vi "motor_controller.vi"() -> ()   [LabVIEW 2020]
panel:
  in  "Crystal Number":u16(ring) items=["Crystal 1", "Crystal 2", "Crystal 3", "Crystal 4", "Crystal 5", "Crystal 6", "Crystal 7", ""]
  in  "Scan speed":dbl
  in  "End":dbl
  in  "Start":dbl
  in  "Start scan":bool
  in  "Tab Control":enum32{"Motor Controls", "Power"}(tab)
  in  "Motor 1":dbl
  in  "Motor 2":dbl
  in  "Motor 3":dbl
  in  "Motor 4":dbl
  in  "Motor 5":dbl
  in  "Motor 6":dbl
  in  "stop":bool
  in  "Motor 7":dbl
  in  "Movement speed":dbl
  in  "Step Size":dbl
  # "Motor Scan"
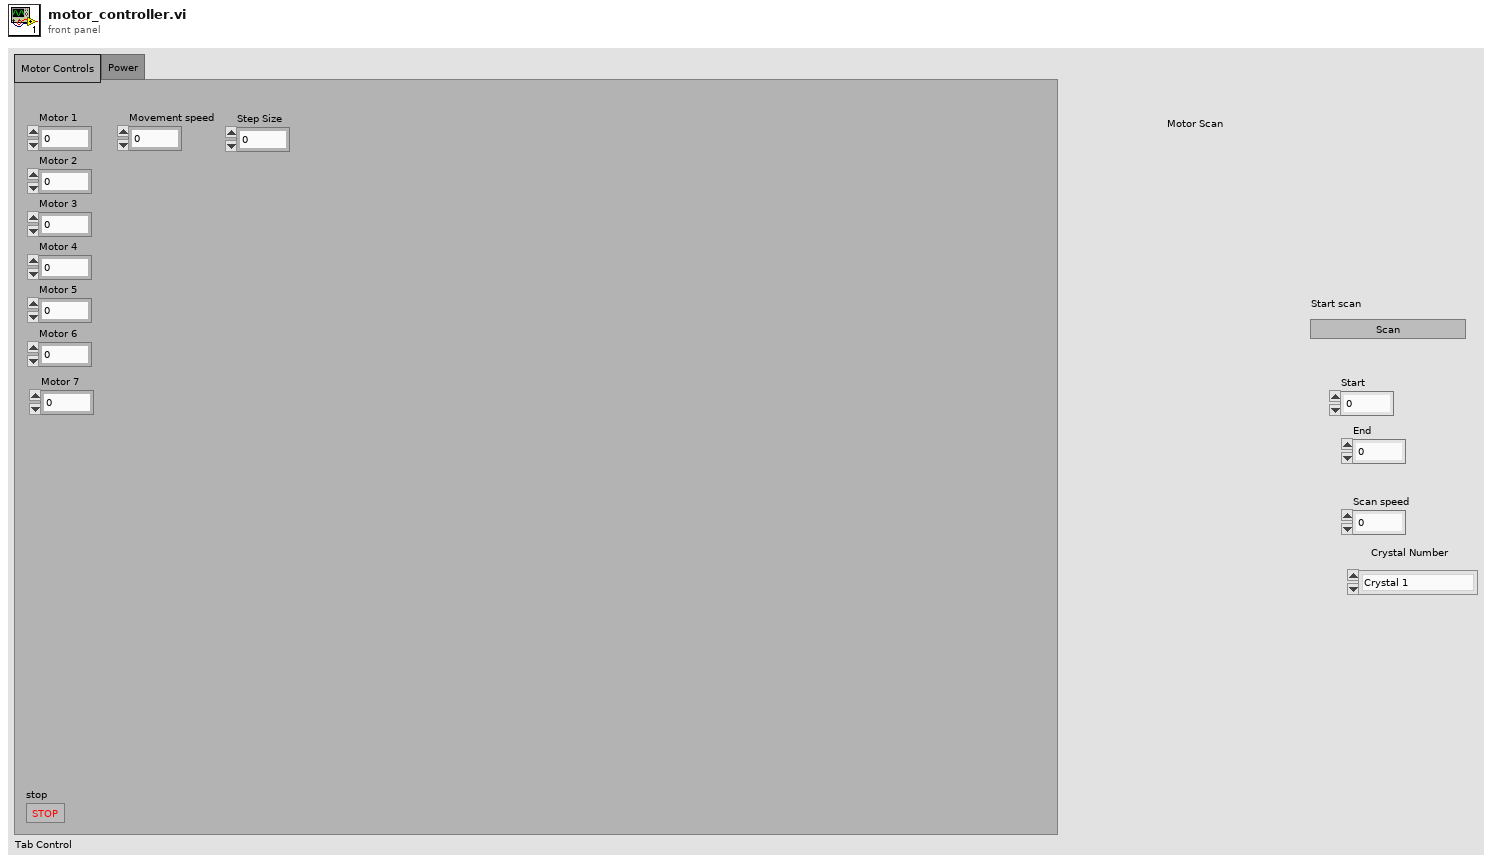
[diagram p1: front panel]
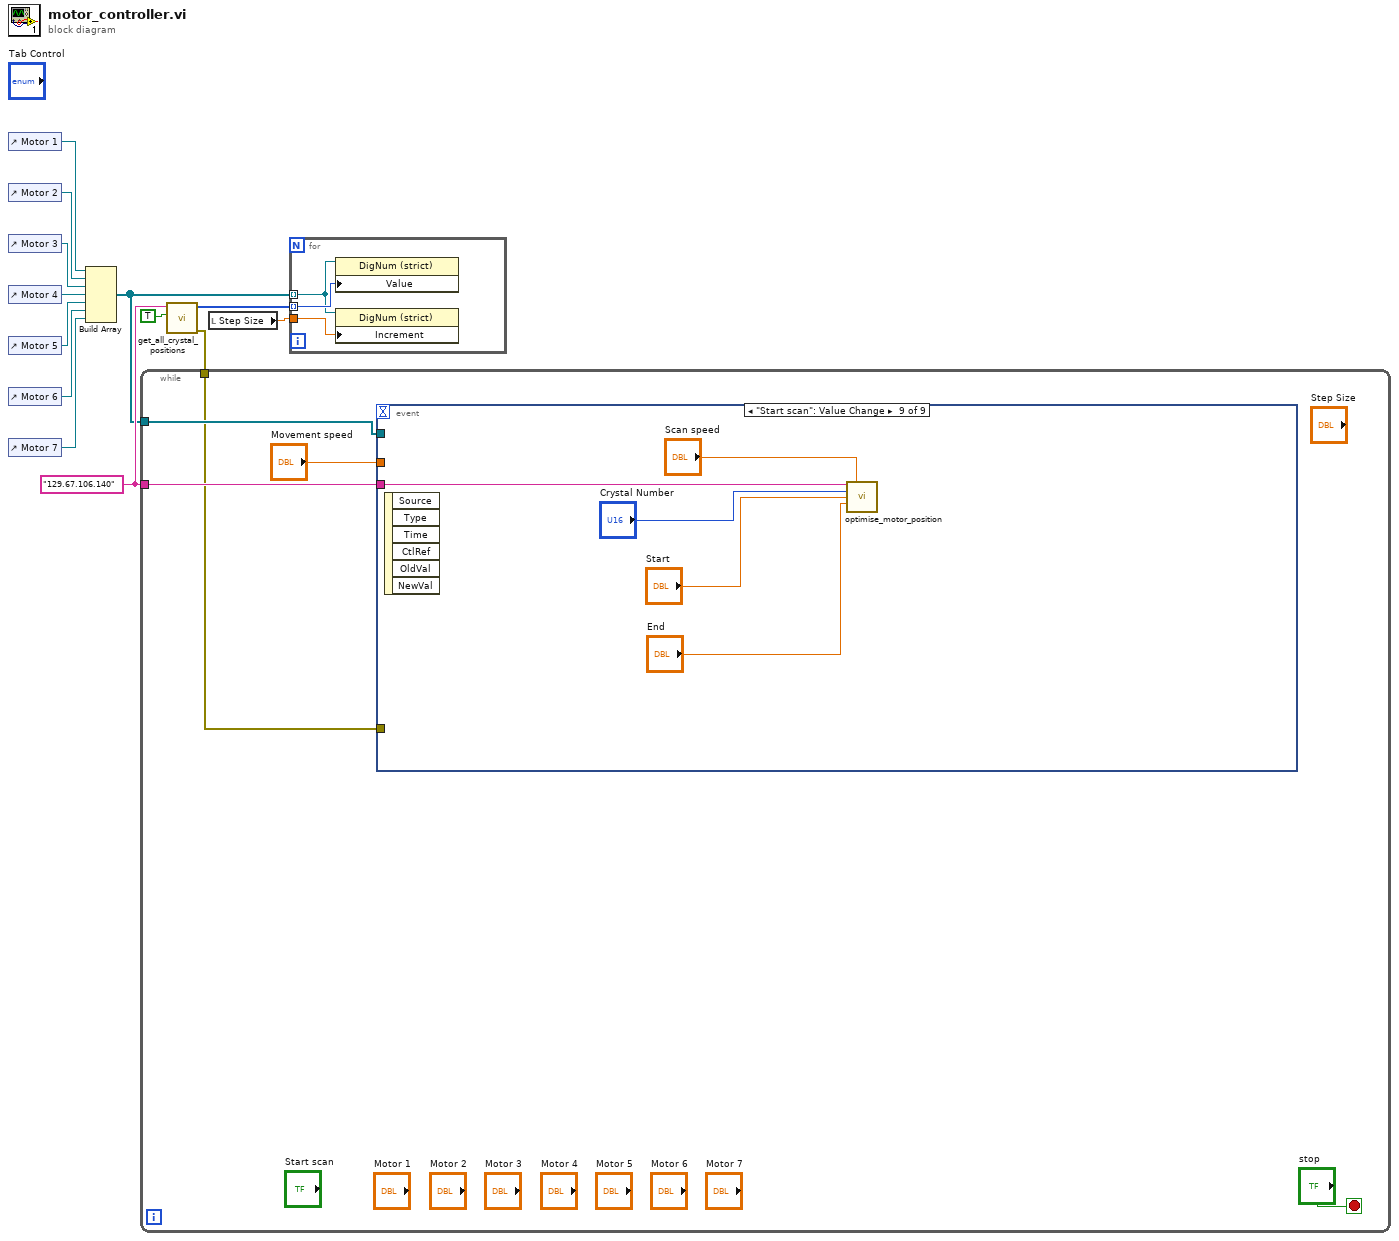
[diagram p0: block diagram]
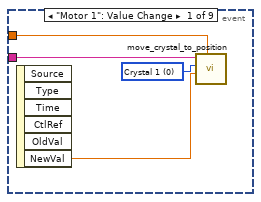
[diagram p2: hidden frame]
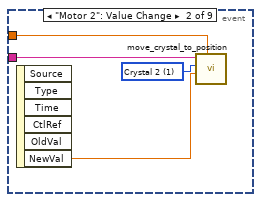
[diagram p3: hidden frame]
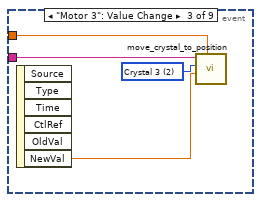
[diagram p4: hidden frame]
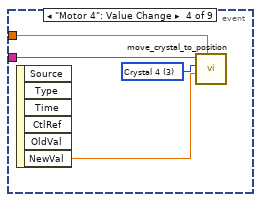
[diagram p5: hidden frame]
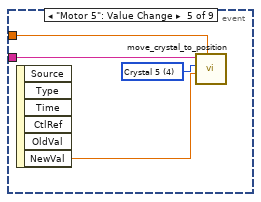
[diagram p6: hidden frame]
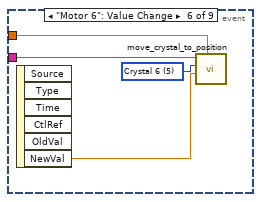
[diagram p7: hidden frame]
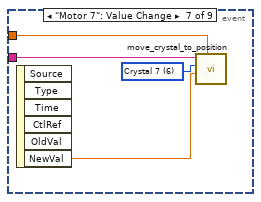
[diagram p8: hidden frame]
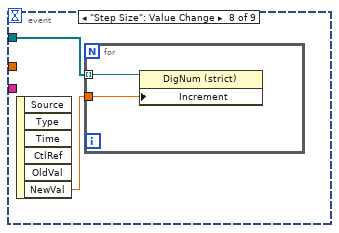
[diagram p9: hidden frame]
diagram:
  w4 = "129.67.106.140" ("address")
  n1 = control-ref of="Motor 1"() -> (w12:refnum<vi>)
  n2 = control-ref of="Motor 2"() -> (w11:refnum<vi>)
  n3 = control-ref of="Motor 3"() -> (w10:refnum<vi>)
  n4 = control-ref of="Motor 4"() -> (w9:refnum<vi>)
  n5 = control-ref of="Motor 5"() -> (w8:refnum<vi>)
  n6 = control-ref of="Motor 6"() -> (w7:refnum<vi>)
  n7 = control-ref of="Motor 7"() -> (w6:refnum<vi>)
  n8 = Build Array(w12, w11, w10, w9, w8, w7, w6) -> (w3:refnum<vi>[])
  n9 = call "get_all_crystal_positions.vi"("7th Crystal?"=TRUE, "address"=w4) -> ("error out"=w1:errorcluster, "Crystal Positions Array"=w5:i32[])  [unwired: 8 in]
  n10 = while {
    tunnel: w4 -> [w17]
    tunnel: w3 -> [w15]
    tunnel: w1 -> [w14]
    stop <- "stop" stop-if-true
    n11 = event shown="[8] \"Start scan\": Value Change" {
      selector: _ -> [_ _ _ _ _ _ _ _ _]
      dyn-events: _ -> [_ _ _ _ _ _ _ _ _]
      timeout: _ -> [_ _ _ _ _ _ _ _ _]
      tunnel: w17 -> [w22 w24 w28 w32 w36 w40 w44 _ w55]
      tunnel: "Movement speed" -> [w19 w23 w27 w31 w35 w39 w43 _ _]
      tunnel: w15 -> [_ _ _ _ _ _ _ w47 _]
      tunnel: w14 -> [_ _ _ _ _ _ _ _ _]
      event "Motor 1": Value Change {
        w21 = u16 0 items=["Crystal 1", "Crystal 2", "Crystal 3", "Crystal 4", "Crystal 5", "Crystal 6", "Crystal 7", ""] ("Crystal Number")
        n12 = event-data() -> ("NewVal"=w20:dbl)  [unwired: 1 in, 5 out]
        n13 = call "move_crystal_to_position.vi"("Crystal Speed / counts s-1"=w19, "Desired Position"=w20, "Crystal Number"=w21, "address"=w22) -> ()  [unwired: 6 in, 2 out]
      }
      event "Motor 2": Value Change {
        w26 = u16 1 items=["Crystal 1", "Crystal 2", "Crystal 3", "Crystal 4", "Crystal 5", "Crystal 6", "Crystal 7", ""] ("Crystal Number")
        n14 = event-data() -> ("NewVal"=w25:dbl)  [unwired: 1 in, 5 out]
        n15 = call "move_crystal_to_position.vi"("Crystal Speed / counts s-1"=w23, "Desired Position"=w25, "Crystal Number"=w26, "address"=w24) -> ()  [unwired: 6 in, 2 out]
      }
      event "Motor 3": Value Change {
        w30 = u16 2 items=["Crystal 1", "Crystal 2", "Crystal 3", "Crystal 4", "Crystal 5", "Crystal 6", "Crystal 7", ""] ("Crystal Number")
        n16 = event-data() -> ("NewVal"=w29:dbl)  [unwired: 1 in, 5 out]
        n17 = call "move_crystal_to_position.vi"("Crystal Speed / counts s-1"=w27, "Desired Position"=w29, "Crystal Number"=w30, "address"=w28) -> ()  [unwired: 6 in, 2 out]
      }
      event "Motor 4": Value Change {
        w34 = u16 3 items=["Crystal 1", "Crystal 2", "Crystal 3", "Crystal 4", "Crystal 5", "Crystal 6", "Crystal 7", ""] ("Crystal Number")
        n18 = event-data() -> ("NewVal"=w33:dbl)  [unwired: 1 in, 5 out]
        n19 = call "move_crystal_to_position.vi"("Crystal Speed / counts s-1"=w31, "Desired Position"=w33, "Crystal Number"=w34, "address"=w32) -> ()  [unwired: 6 in, 2 out]
      }
      event "Motor 5": Value Change {
        w38 = u16 4 items=["Crystal 1", "Crystal 2", "Crystal 3", "Crystal 4", "Crystal 5", "Crystal 6", "Crystal 7", ""] ("Crystal Number")
        n20 = event-data() -> ("NewVal"=w37:dbl)  [unwired: 1 in, 5 out]
        n21 = call "move_crystal_to_position.vi"("Crystal Speed / counts s-1"=w35, "Desired Position"=w37, "Crystal Number"=w38, "address"=w36) -> ()  [unwired: 6 in, 2 out]
      }
      event "Motor 6": Value Change {
        w42 = u16 5 items=["Crystal 1", "Crystal 2", "Crystal 3", "Crystal 4", "Crystal 5", "Crystal 6", "Crystal 7", ""] ("Crystal Number")
        n22 = event-data() -> ("NewVal"=w41:dbl)  [unwired: 1 in, 5 out]
        n23 = call "move_crystal_to_position.vi"("Crystal Speed / counts s-1"=w39, "Desired Position"=w41, "Crystal Number"=w42, "address"=w40) -> ()  [unwired: 6 in, 2 out]
      }
      event "Motor 7": Value Change {
        w46 = u16 6 items=["Crystal 1", "Crystal 2", "Crystal 3", "Crystal 4", "Crystal 5", "Crystal 6", "Crystal 7", ""] ("Crystal Number")
        n24 = event-data() -> ("NewVal"=w45:dbl)  [unwired: 1 in, 5 out]
        n25 = call "move_crystal_to_position.vi"("Crystal Speed / counts s-1"=w43, "Desired Position"=w45, "Crystal Number"=w46, "address"=w44) -> ()  [unwired: 6 in, 2 out]
      }
      event "Step Size": Value Change {
        n26 = event-data() -> ("NewVal"=w48:dbl)  [unwired: 1 in, 5 out]
        n27 = for {
          tunnel: w48 -> [w50]
          tunnel: w47 -> [w49] mode=indexing
          n28 = property class="DigNum (strict)"(reference=w49, "Increment"=w50) -> ()  [unwired: 1 in, 2 out]
        }
      }
      event "Start scan": Value Change {
        n29 = event-data() -> ()  [unwired: 1 in, 6 out]
        n30 = call "optimise_motor_position.vi"("address"=w55, "Crystal Speed / counts s-1"="Scan speed", "Crystal Number"="Crystal Number", "Start Position"="Start", "End Position"="End") -> ()  [unwired: 9 in, 2 out]
      }
    }
  }
  n31 = local read "Step Size"() -> (w2:dbl)
  n32 = for {
    tunnel: w3 -> [w57] mode=indexing
    tunnel: w5 -> [w58] mode=indexing
    tunnel: w2 -> [w56]
    n33 = property class="DigNum (strict)"(reference=w57, "Value"=w58) -> ()  [unwired: 1 in, 2 out]
    n34 = property class="DigNum (strict)"(reference=w57, "Increment"=w56) -> ()  [unwired: 1 in, 2 out]
  }
